vi "WSVCAP SHL Host LL RFFE Set Read_Write Parameters.vi"(0 "Transaction":T2=enum."RFFE-Ext Write", 1 "Slave Address":u8, 5 "Wait Ticks":u32, 7 "Bytes to Write":u8, 9 "Socket Mask [U64]":u64 format="%04x", 11 "error in (no error)":errorcluster, 12 "Sub Address (Ext-Read Only)":u16 format="%04x", 13 "Bytes to Read (Ext-Read Only)":u8 format="%04x", 14 "FPGA":T1) -> (15 "error out":errorcluster)   [LabVIEW 2017]
uses:
  Type Defs/WSVCAP SHL Transaction Enum.ctl
  Type Defs/WSVCAP SHL FPGA Enum.ctl
  Type Defs/WSVCAP SHL Top Level Control Operation Enum.ctl
  Type Defs/WSVCAP SHL State.ctl
  Type Defs/WSVCAP SHL Top Level Control Enum.ctl
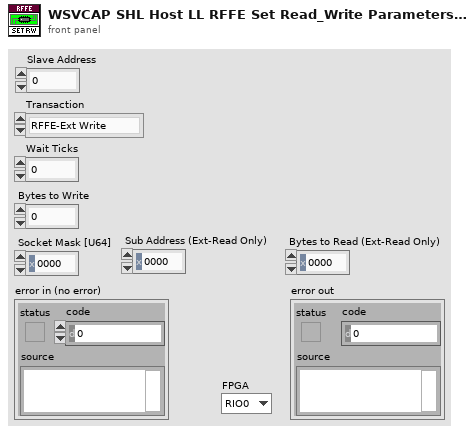
[diagram p1: front panel]
types:
  T1 = typedef "WSVCAP SHL FPGA Enum.ctl" = enum16{"RIO0", "RIO1"}
  T2 = typedef "WSVCAP SHL Transaction Enum.ctl" = enum16{"I2C-Read Data", "I2C-Write Data", "RFFE-Ext Write", "RFFE-Ext Read"}
  T3 = typedef "WSVCAP SHL Top Level Control Operation Enum.ctl" = enum16{"Initialize", "Set Control", "Read Control", "Close"}
  T4 = typedef "WSVCAP SHL State.ctl" = enum8{"Idle", "Transfer Data"}
  T5 = typedef "WSVCAP SHL Top Level Control Enum.ctl" = enum16{"Start", "Cmd", "Transaction", "Wait Ticks", "Socket Mask", "UUT Set", "Slave Address", "Sub Address", "Bytes to Write", "Bytes to Read", "Write Data", "Write Flag", "Read Data", "Read Flag", "Ack Read", "Read Status Flag", "Ack Read Status", "Status", "Cycle Count", "Stop Cycle", "Exit"}
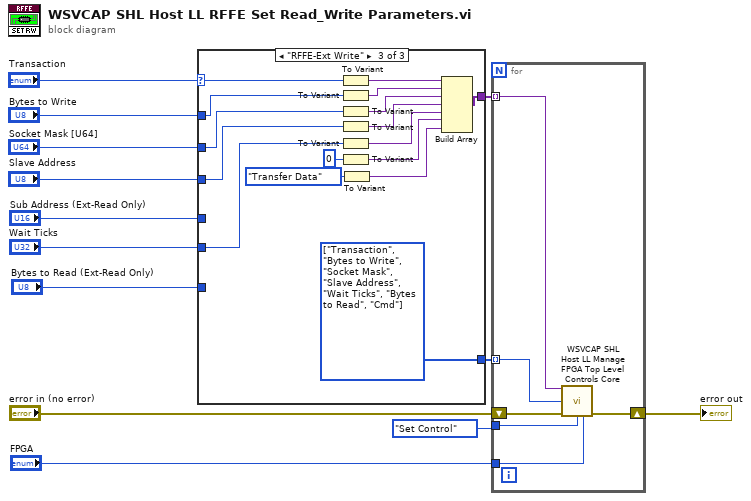
[diagram p0: block diagram]
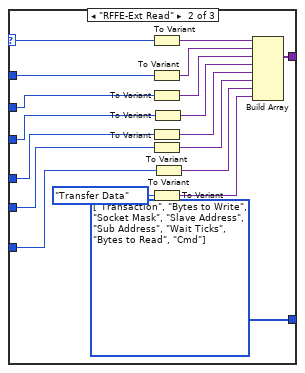
[diagram p3: hidden frame]
diagram:
  n1 = case shown="\"RFFE-Ext Write\"" "Transaction" {
    selector: "Transaction" -> [_ w20 w36]
    tunnel: [_ w28 w44] -> w12
    tunnel: [_ w26 w42] -> w9
    tunnel: "Socket Mask [U64]" -> [_ w25 w41]
    tunnel: "Bytes to Write" -> [_ w23 w39]
    tunnel: "Wait Ticks" -> [_ w22 w38]
    tunnel: "Sub Address (Ext-Read Only)" -> [_ w19 _]
    tunnel: "Slave Address" -> [_ w17 w35]
    tunnel: "Bytes to Read (Ext-Read Only)" -> [_ w15 _]
    frame Default {
    }
    frame "RFFE-Ext Read" {
      w26 = T5[] [enum."Transaction", enum."Bytes to Write", enum."Socket Mask", enum."Slave Address", enum."Sub Address", enum."Wait Ticks", enum."Bytes to Read", enum."Cmd"] items=["Start", "Cmd", "Transaction", "Wait Ticks", "Socket Mask", "UUT Set", "Slave Address", "Sub Address", "Bytes to Write", "Bytes to Read", "Write Data", "Write Flag", "Read Data", "Read Flag", "Ack Read", "Read Status Flag", "Ack Read Status", "Status", "Cycle Count", "Stop Cycle", "Exit"]
      n2 = To Variant(anything=w20) -> (Variant=w30:variant)
      n3 = To Variant(anything=w23) -> (Variant=w29:variant)
      n4 = To Variant(anything=w25) -> (Variant=w24:variant)
      n5 = To Variant(anything=w19) -> (Variant=w18:variant)
      n6 = To Variant(anything=w22) -> (Variant=w21:variant)
      n7 = To Variant(anything=WSVCAP_SHL_State."Transfer Data" ("SPI_Cmd")) -> (Variant=w27:variant)
      n8 = To Variant(anything=w17) -> (Variant=w16:variant)
      n9 = To Variant(anything=w15) -> (Variant=w14:variant)
      n10 = Build Array(w30, w29, w24, w16, w18, w21, w14, w27) -> (w28:variant[])
    }
    frame "RFFE-Ext Write" {
      w42 = T5[] [enum."Transaction", enum."Bytes to Write", enum."Socket Mask", enum."Slave Address", enum."Wait Ticks", enum."Bytes to Read", enum."Cmd"] items=["Start", "Cmd", "Transaction", "Wait Ticks", "Socket Mask", "UUT Set", "Slave Address", "Sub Address", "Bytes to Write", "Bytes to Read", "Write Data", "Write Flag", "Read Data", "Read Flag", "Ack Read", "Read Status Flag", "Ack Read Status", "Status", "Cycle Count", "Stop Cycle", "Exit"]
      n11 = To Variant(anything=w36) -> (Variant=w46:variant)
      n12 = To Variant(anything=w39) -> (Variant=w45:variant)
      n13 = To Variant(anything=w41) -> (Variant=w40:variant)
      n14 = To Variant(anything=w35) -> (Variant=w34:variant)
      n15 = To Variant(anything=w38) -> (Variant=w37:variant)
      n16 = To Variant(anything=u8 0 ("Bytes to Read (Ext-Read Only)")) -> (Variant=w33:variant)
      n17 = To Variant(anything=WSVCAP_SHL_State."Transfer Data" ("SPI_Cmd")) -> (Variant=w43:variant)
      n18 = Build Array(w46, w45, w40, w34, w37, w33, w43) -> (w44:variant[])
    }
  }
  n19 = for {
    tunnel: WSVCAP_SHL_Top_Level_Control_Operation_Enum."Set Control" ("Operation") -> [w53]
    tunnel: w12 -> [w52] mode=indexing
    tunnel: w9 -> [w51] mode=indexing
    shift-right: [w49] -> w10
    shift-left: "error in (no error)" -> [w50]
    tunnel: "FPGA" -> [w48]
    n20 = call "WSVCAP SHL Host LL Manage FPGA Top Level Controls Core.vi"("Value In"=w52, "FPGA Top Level Control"=w51, "error in (no error)"=w50, "Operation"=w53, "FPGA"=w48) -> ("error out"=w49:errorcluster)  [unwired: 9 in, 1 out]
  }
  "error out" <- w10
